vi "Build Resistor Ciphers.vi"(7 "Number of Bands":T3=4 min=3 max=6 step=1, 8 "error in (no error)":errorcluster, 11 "Resistance Digits":T1) -> (0 "error out":errorcluster, 2 "Negative":bool, 3 "Nominal Value":i32)   [LabVIEW 2018]
doc: "Builds the Ciphers array used to calculate the resistor significant value according to the selected number of bands.\n\nThe VI receives the <b>Number of Bands</b> and the resistor significant digits through <b>MSD Digit</b>, <b>MID Digit</b>, and <b>LSD Digit</b> inside the cluster <b>Resistance Digits</b>.\n\nFor 3- and 4-band resistors, the resistor has two significant digits. The resulting Ciphers array is built as:\n\n[0, MSD Digit, LSD Digit]\n\nFor 5- and 6-band resistors, the resistor has three significant digits. The resulting Ciphers array is built as:\n\n[MSD Digit, MID Digit, LSD Digit]\n\nThe resulting Ciphers array is intended to be passed to <b>Cipher to Number.vi</b>."
uses:
  Number of Bands--number.ctl
  Resistance Digits--cluster.ctl
  Digit--enum.ctl
panel:
  # "LSD = Least Significant Digit)"
  # "Middle Digit"
  # "MSD = Most Significant Digit"
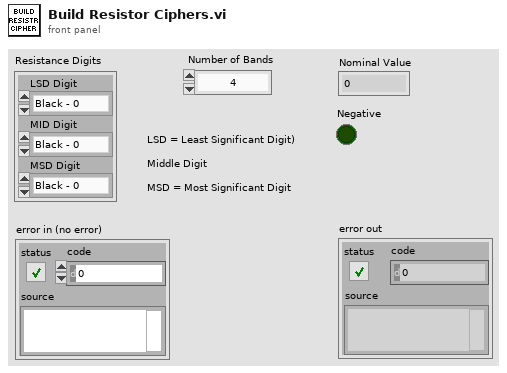
[diagram p1: front panel]
types:
  T1 = typedef "Resistance Digits--cluster.ctl" = cluster{"LSD Digit":T2, "MID Digit":T2, "MSD Digit":T2}
  T2 = typedef "digit--enum.ctl" = enum16{"Black - 0", "Brown - 1", "Red - 2", "Orange - 3", "Yellow - 4", "Green - 5", "Blue - 6", "Violet - 7", "Grey - 8", "White - 9"}
  T3 = typedef "Number of Bands--number.ctl" = u8
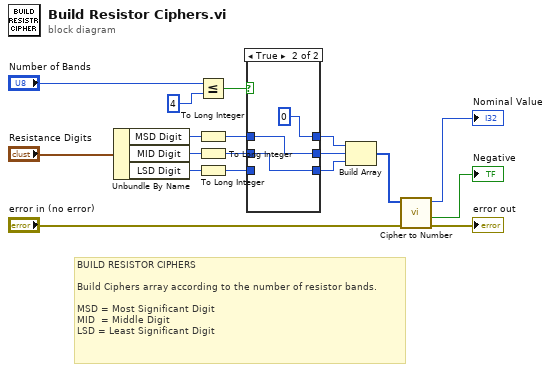
[diagram p0: block diagram]
diagram:
  # "BUILD RESISTOR CIPHERS\n\nBuild Ciphers array according to the number of resistor bands.\n\nMSD = Most Significant Digit\nMID  = Middle Digit\nLSD = Least Significant Digit"
  n1 = Unbundle By Name("Resistance Digits") -> ("MSD Digit"=w10:T2, "MID Digit"=w9:T2, "LSD Digit"=w8:T2)
  n2 = Less Or Equal?(x="Number of Bands", y=T3 4) -> (x <= y?=w7:bool)
  n3 = To Long Integer(number=w10) -> (32bit integer=w6:i32)
  n4 = To Long Integer(number=w9) -> (32bit integer=w5:i32)
  n5 = To Long Integer(number=w8) -> (32bit integer=w4:i32)
  n6 = case shown="True" w7 {
    tunnel: w6 -> [w21 w23]
    tunnel: w5 -> [w20 w24]
    tunnel: w4 -> [w19 _]
    tunnel: [w21 0] -> w3
    tunnel: [w20 w23] -> w2
    tunnel: [w19 w24] -> w1
    frame False {
    }
    frame True {
    }
  }
  n7 = Build Array(w3, w2, w1) -> (w12:i32[])
  n8 = call "Cipher to Number.vi"("error in (no error)"="error in (no error)", "Ciphers"=w12) -> ("error out"=→"error out":errorcluster, "Negative"=→"Negative":bool, "Number"=→"Nominal Value":i32)  [unwired: 7 in]
